vi "DSF.Engine.Plugin.Get Transceiver Thread.vi"(10 "index":i32, 11 "Plugin in":refnum<class "DSF.Engine.Plugin.lvclass">) -> (2 "Transceiver Thread":refnum<class "DSF.Engine.Interface.Transceiver.lvclass">, 3 "Plugin out":refnum<class "DSF.Engine.Plugin.lvclass">)   [LabVIEW 2017, in "DSF.Engine.lvlib" / "DSF.Engine.Plugin.lvclass"]
uses:
  DSF.Engine.Plugin.lvclass
  Interface/DSF.Engine.Interface.Transceiver.lvclass
  DSF.Engine.Plugin.lvclass/DSF.Engine.Plugin.ctl
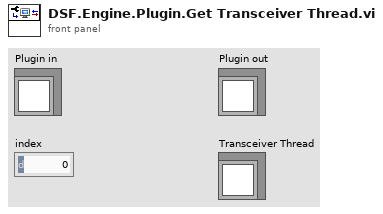
[diagram p1: front panel]
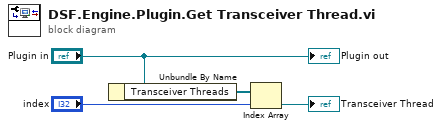
[diagram p0: block diagram]
diagram:
  n1 = Unbundle By Name("Plugin in") -> ("Transceiver Threads"=w3:refnum<class "DSF.Engine.Interface.Transceiver.lvclass">[])
  n2 = Index Array(array=w3, index="index") -> (element=→"Transceiver Thread":refnum<class "DSF.Engine.Interface.Transceiver.lvclass">)
  "Plugin out" <- "Plugin in"
